vi "Sequence.FormatConditions.vi"(4 "Aliases.All":T3[](array[typedef]), 6 "Aliases Array":string[](array[string]), 8 "error in (no error)":errorcluster, 10 "Conditions":string[](array[string]), 11 "variant in":variant) -> (0 "error out":errorcluster, 1 "Warning":string, 2 "Condition":T1={"First Opreation"=enum."||", "Expression"=""}, 3 "variant out":variant)   [LabVIEW 2013, in "Simple Sequence Tools - Editor.lvlib"]
uses:
  Simple Sequence Tools - Editor.lvlib
  Shared/Types/ChannelProperties.ctl
  Types/Compiled.StepCondition.ctl
  Types/OperationTypes.ctl
  C:/Program Files/National Instruments/VeriStand 2013/Data/NationalInstruments.VeriStand.RealTimeSequenceDefinitionApiUtilities.dll
  Program Files/National Instruments/VeriStand 2013/Data/NationalInstruments.VeriStand.RealTimeSequenceDefinitionApiUtilities.dll
  Shared/Simple Sequence Tools - Shared.lvlib
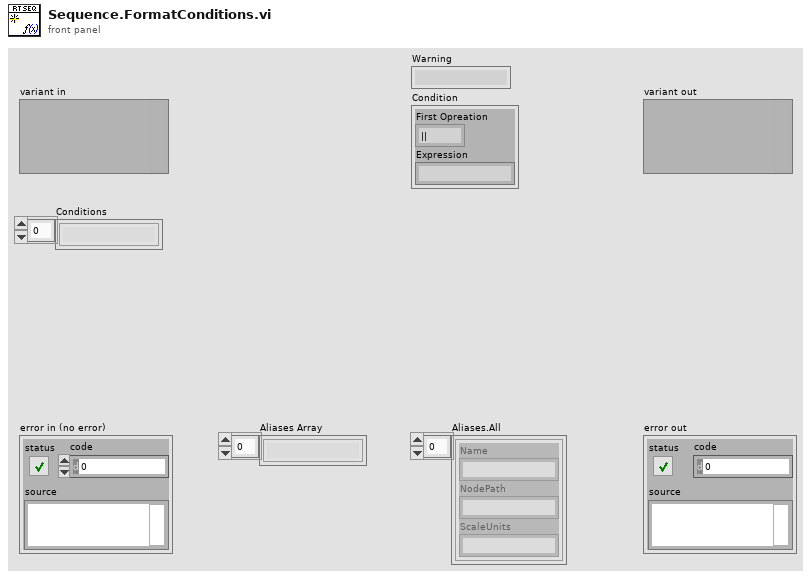
[diagram p1: front panel]
types:
  T1 = typedef "Simple Sequence Tools - Editor.lvlib/Compiled.StepCondition.ctl" = cluster{"First Opreation":T2, "Expression":string}
  T2 = typedef "Simple Sequence Tools - Editor.lvlib/OperationTypes.ctl" = enum8{"None", "&&", "||"}
  T3 = typedef "Simple Sequence Tools - Shared.lvlib/ChannelProperties.ctl" = cluster{"Name":string, "NodePath":string, "ScaleUnits":string}
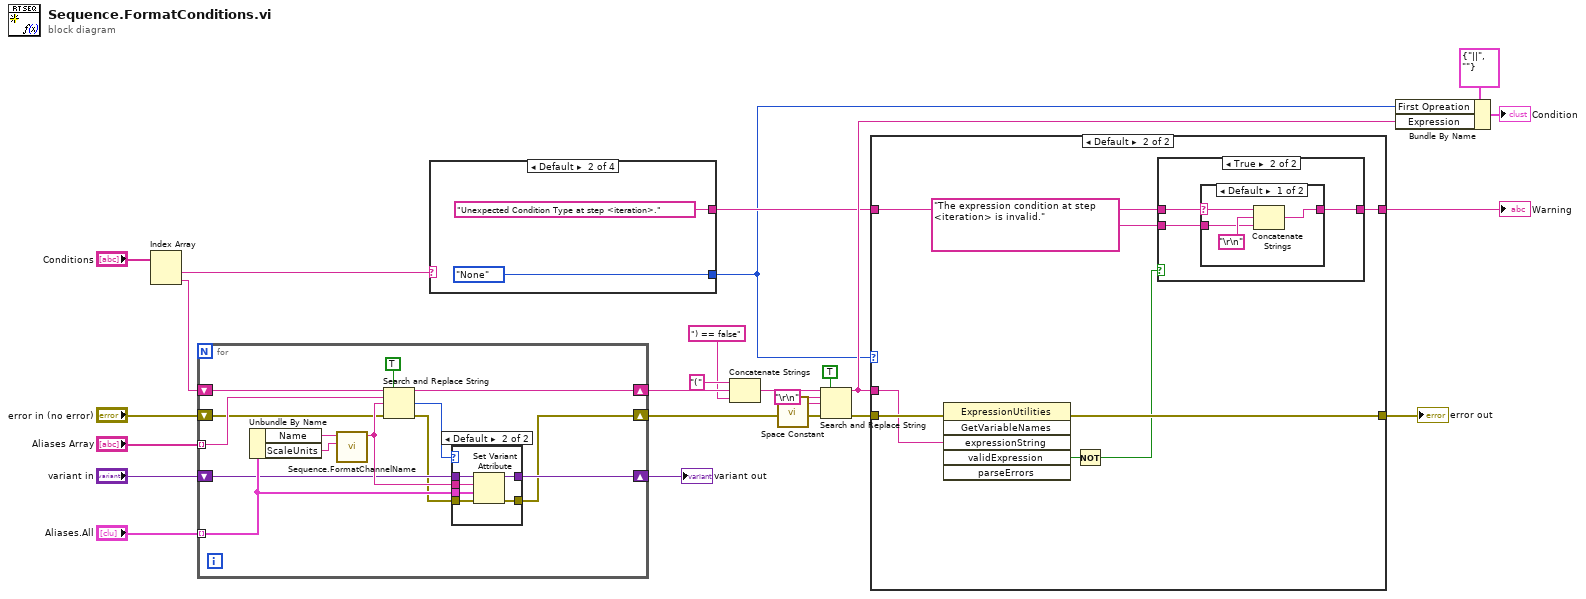
[diagram p0: block diagram]
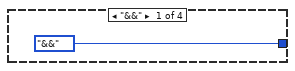
[diagram p6: hidden frame]
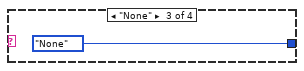
[diagram p7: hidden frame]
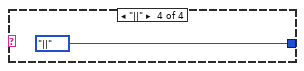
[diagram p8: hidden frame]
diagram:
  n1 = Index Array(array="Conditions") -> (element #1=w12:string, element #2=w11:string)  [unwired: 2 in]
  n2 = for {
    tunnel: "Aliases Array" -> [w38] mode=indexing
    tunnel: "Aliases.All" -> [w32] mode=indexing
    shift-right: [w25] -> w21
    shift-left: "error in (no error)" -> [w29]
    shift-right: [w33] -> w10
    shift-left: w11 -> [w37]
    shift-right: [w30] -> w24
    shift-left: "variant in" -> [w27]
    n3 = Unbundle By Name(w32) -> ("Name"=w35:string, "ScaleUnits"=w36:string)
    n4 = call "Sequence.FormatChannelName.vi"("ScaleUnits"=w36, "Name"=w35) -> ("ChannelName"=w31:string)  [unwired: 9 in]
    n5 = Search and Replace String(replace all?=TRUE ("replace all? (F)"), input string=w37, search string=w38, replace string=w31, error in=w29) -> (result string=w33:string, number of replacements=w28:i32, error out=w26:errorcluster)  [unwired: 3 in, 1 out]
    n6 = case shown="Default" w28 {
      tunnel: w32 -> [_ w46]
      tunnel: w31 -> [_ w45]
      tunnel: [w40 w44] -> w30
      tunnel: w27 -> [w40 w43]
      tunnel: w26 -> [w39 w42]
      tunnel: [w39 w41] -> w25
      frame -1, 0 {
      }
      frame Default {
        n7 = Set Variant Attribute(Variant=w43, name=w45, value=w46, error in=w42) -> (Variant out=w44:variant, error out=w41:errorcluster)  [unwired: 1 out]
      }
    }
  }
  "variant out" <- w24
  n8 = case shown="Default" w12 {
    tunnel: [OperationTypes."&&" OperationTypes."None" OperationTypes."None" OperationTypes."||"] -> w2
    tunnel: [_ "Unexpected Condition Type at step <iteration>." _ _] -> w4
    frame "&&" {
    }
    frame Default {
    }
    frame "None" {
    }
    frame "||" {
    }
  }
  n9 = Concatenate Strings("(" ("string"), w10, ") == false" ("string")) -> (w18:string)
  n10 = call <vilib>:"Space Constant.vi"() -> ("String"=w20:string)
  n11 = Search and Replace String(replace all?=TRUE ("replace all? (F)"), input string=w18, search string="\r\n", replace string=w20, error in=w21) -> (result string=w5:string, error out=w6:errorcluster)  [unwired: 3 in, 2 out]
  n12 = case shown="Default" w2 {
    tunnel: w6 -> [w52 w61]
    tunnel: w5 -> [_ w55]
    tunnel: w4 -> [w53 w59]
    tunnel: [w53 w58] -> w3
    tunnel: [w52 w57] -> w1
    frame "None" {
    }
    frame Default {
      n13 = invoke class="ExpressionUtilities" method="GetVariableNames"(error in=w61, "expressionString"=w55) -> (error out=w57:errorcluster, "validExpression"=w60:bool)  [unwired: 4 in, 4 out]
      n14 = Not(x=w60) -> (.not. x?=w54:bool)
      n15 = case shown="True" w54 {
        tunnel: w59 -> [w62 w64]
        tunnel: [w62 w65] -> w58
        tunnel: "The expression condition at step <iteration> is invalid." ("result string") -> [_ w63]
        frame False {
        }
        frame True {
          n16 = case shown="Default" w64 {
            selector: w64 -> [w69 _]
            tunnel: [w67 w70] -> w65
            tunnel: w63 -> [w66 w70]
            frame Default {
              n17 = Concatenate Strings(w69, "\r\n", w66) -> (w67:string)
            }
            frame "" {
            }
          }
        }
      }
    }
  }
  "Warning" <- w3
  "error out" <- w1
  n18 = Bundle By Name(cluster=T1 {"First Opreation"=enum."||", "Expression"=""} ("Condition"), "First Opreation"=w2, "Expression"=w5) -> (→"Condition":T1)
